vi "Get Frame from TDMS.vi"(6 "Channel Name(s)":string[](array[string]), 9 "Frame Number":i32, 10 "base path":path, 11 "TDMS Ref":refnum<k34>) -> (2 "Paths for TIFFs":path[](array[path]), 3 "tdms file out":refnum<k34>, 5 "pDataBuffer":u16[](array[numeric]))   [LabVIEW 2020]
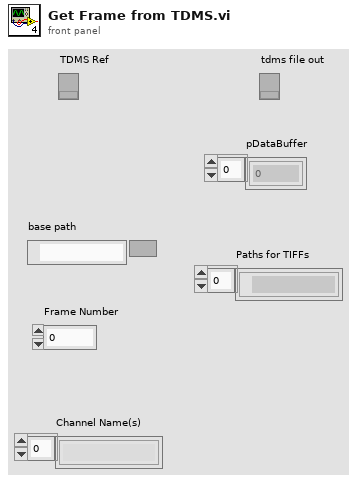
[diagram p1: front panel]
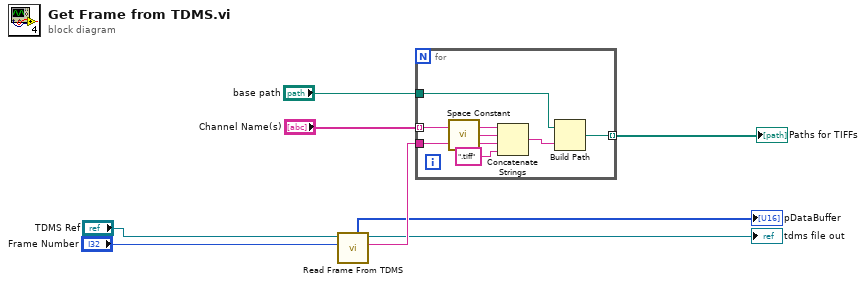
[diagram p0: block diagram]
diagram:
  n1 = call "Read Frame From TDMS.vi"("Frame Number"="Frame Number", "tdms file in"="TDMS Ref") -> ("\"frame n\" string"=w3:string, "tdms file out"=→"tdms file out":refnum<k34>, "pDataBuffer"=→"pDataBuffer":u16[])  [unwired: 7 in]
  n2 = for {
    tunnel: "Channel Name(s)" -> [w11] mode=indexing
    tunnel: "base path" -> [w13]
    tunnel: [w12] -> w4 mode=indexing
    tunnel: w3 -> [w10]
    n3 = call <vilib>:"Space Constant.vi"() -> ("String"=w9:string)
    n4 = Concatenate Strings(w11, w9, w10, ".tiff" ("string")) -> (w14:string)
    n5 = Build Path(base path=w13, name or relative path=w14) -> (appended path=w12:path)
  }
  "Paths for TIFFs" <- w4
